vi "ЛР1 -  варик.vi"() -> ()   [LabVIEW 2012]
panel:
  out "фунт-сила на кв. дюйм":dbl(slide) scale=-60.0..130.0
  in  "мм.рт.ст./\nфунт-сила\nна кв. дюйм":bool
  out "мм.рт.ст":dbl(slide) scale=-60.0..130.0
  in  "Паскаль":dbl(slide) scale=-50.0..50.0
  # "Паскаль"
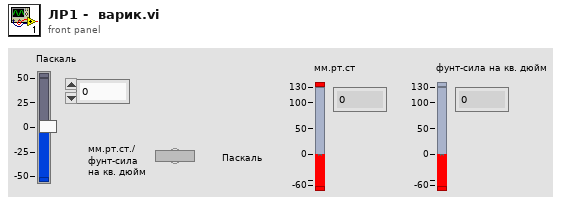
[diagram p1: front panel]
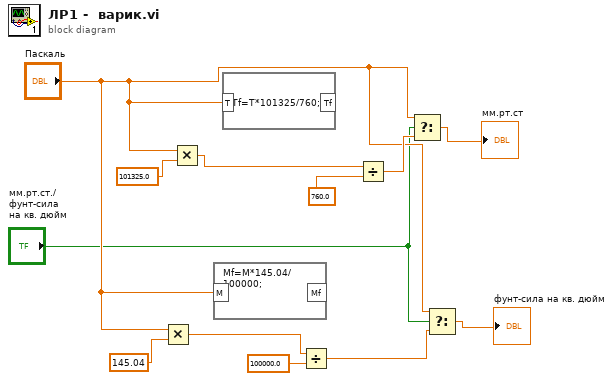
[diagram p0: block diagram]
diagram:
  n1 = Multiply(x="Паскаль", y=145.04) -> (x*y=w6:dbl)
  n2 = Multiply(x="Паскаль", y=101325.0) -> (x*y=w8:dbl)
  n3 = formula code="Mf=M*145.04/100000;"("M"="Паскаль") -> ()  [unwired: 1 out]
  n4 = formula code="Tf=T*101325/760;"("T"="Паскаль") -> ()  [unwired: 1 out]
  n5 = Divide(x=w6, y=100000.0) -> (x/y=w4:dbl)
  n6 = Divide(x=w8, y=760.0) -> (x/y=w3:dbl)
  n7 = Select(t="Паскаль", s="мм.рт.ст./\nфунт-сила\nна кв. дюйм", f=w3) -> (s? t:f=→"мм.рт.ст":dbl)
  n8 = Select(t="Паскаль", s="мм.рт.ст./\nфунт-сила\nна кв. дюйм", f=w4) -> (s? t:f=→"фунт-сила на кв. дюйм":dbl)
